vi "LS218_WRITE_ETAT_VOIE.vi"(4 "numéro voie":i32, 5 "entrée d'erreur (pas d'erreur)":errorcluster, 6 "INPUT ON":bool, 7 "Input_curve":u16(ring)=6 items=["aucune", "DT-470 (diode)", "DT-500 (diode)", "CTI (diode)", "DT- 670 (diode)", "Cernox", "Pt100", "Pt1000"], 8 "Refnum VISA en entrée":refnum<visa-resource-name>) -> (0 "sortie d'erreur":errorcluster, 3 "Nom de ressource VISA en sortie":refnum<visa-resource-name>)   [LabVIEW 2016]
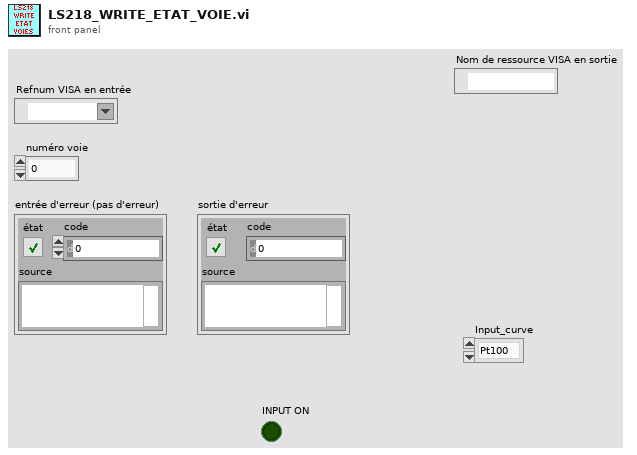
[diagram p1: front panel]
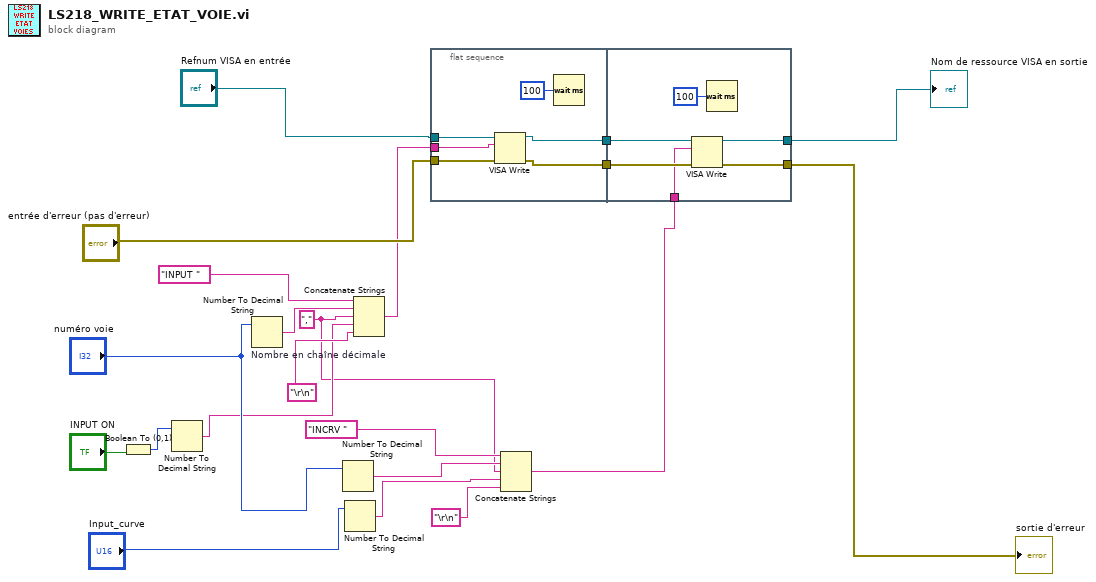
[diagram p0: block diagram]
diagram:
  w10 = "," ("chaîne")
  n1 = Boolean To (0,1)(Boolean="INPUT ON") -> (0, 1=w15:i16)
  n2 = Number To Decimal String ("Nombre en chaîne décimale")(number=w15) -> (decimal integer string=w13:string)  [unwired: 1 in]
  n3 = Number To Decimal String "Nombre en chaîne décimale"(number="numéro voie") -> (decimal integer string=w21:string)  [unwired: 1 in]
  n4 = Number To Decimal String(number="numéro voie") -> (decimal integer string=w18:string)  [unwired: 1 in]
  n5 = Number To Decimal String(number="Input_curve") -> (decimal integer string=w11:string)  [unwired: 1 in]
  n6 = Concatenate Strings("INPUT " ("chaîne"), w21, w10, w13, "\r\n" ("chaîne")) -> (w6:string)
  n7 = flat-sequence {
    tunnel: "Refnum VISA en entrée" -> [w27]
    tunnel: "entrée d'erreur (pas d'erreur)" -> [w26]
    tunnel: w6 -> [w25]
    tunnel: [w24] -> w5
    tunnel: [w23] -> w4
    tunnel: w5 -> [w33]
    tunnel: w4 -> [w32]
    tunnel: w3 -> [w31]
    tunnel: [w30] -> w2
    tunnel: [w29] -> w1
    frame #0 {
      n8 = VISA Write(VISA resource name=w27, write buffer=w25, error in (no error)=w26) -> (VISA resource name out=w23:refnum<visa-resource-name>, error out=w24:errorcluster)  [unwired: 1 out]
      n9 = Wait (ms)(milliseconds to wait=u32 100 ("attente (ms)")) -> ()  [unwired: 1 out]
    }
    frame #1 {
      n10 = VISA Write(VISA resource name=w32, write buffer=w31, error in (no error)=w33) -> (VISA resource name out=w30:refnum<visa-resource-name>, error out=w29:errorcluster)  [unwired: 1 out]
      n11 = Wait (ms)(milliseconds to wait=u32 100 ("attente (ms)")) -> ()  [unwired: 1 out]
    }
  }
  n12 = Concatenate Strings("INCRV " ("chaîne"), w18, w10, w11, "\r\n" ("chaîne")) -> (w3:string)
  "sortie d'erreur" <- w1
  "Nom de ressource VISA en sortie" <- w2
